vi "Model - DeInit.vi"(8 "error in (no error)":errorcluster, 11 "View Model":T1) -> (0 "error out":errorcluster)   [LabVIEW 2017]
doc: "Deletes all DVR and Destroy all user events from View Model"
uses:
  Controls/View Model.ctl
  Configuration Database/Controls/Config Model.ctl
  Configuration Database/Controls/Config Commands.ctl
  Configuration Database/Controls/Congif Data.ctl
  Controls/Shared Model.ctl
  Error Handler/Controls/Error Model.ctl
  Error Handler/Controls/Error Data.ctl
  Error Handler/Controls/Error Type.ctl
  Car Wash Controller/Controls/Car Wash Model.ctl
  Car Wash Controller/Controls/Controller Overhead.ctl
  Car Wash Controller/Controls/Vehicle Location.ctl
  Car Wash Controller/Controls/Car Wash States.ctl
  Car Wash Controller/Controls/CarWash CMD.ctl
  Views/Wash Display Console View/Controls/Car Wash Indicators.ctl
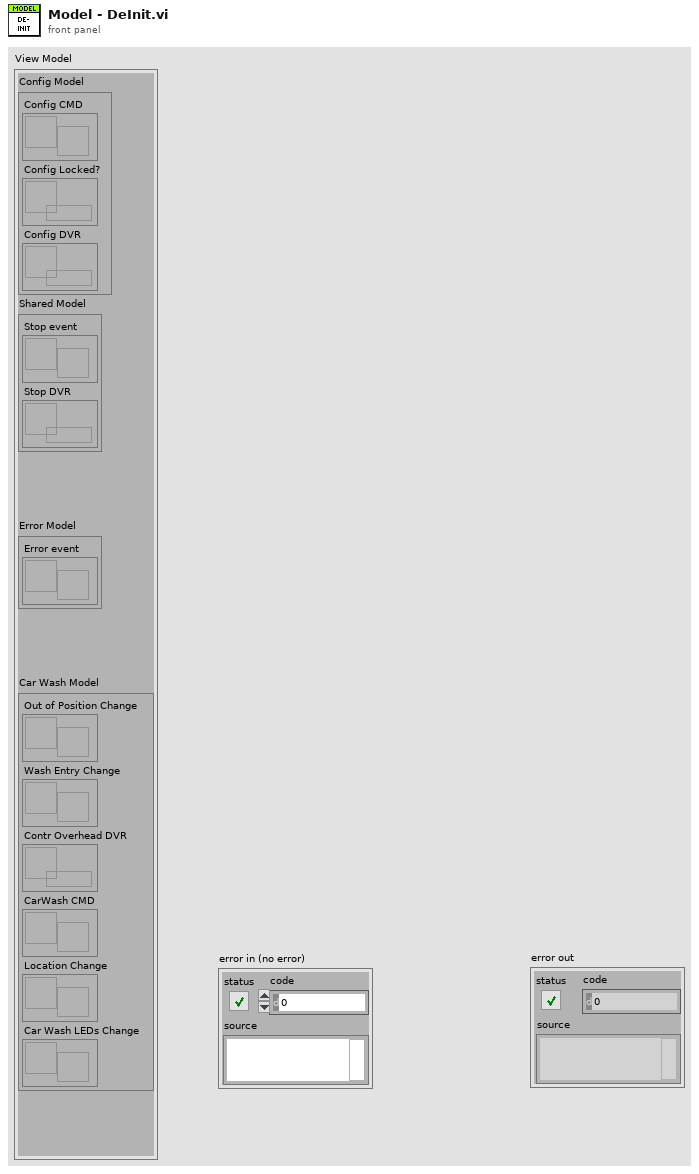
[diagram p1: front panel]
types:
  T1 = typedef "View Model.ctl" = cluster{"Config Model":T2, "Shared Model":T3, "Error Model":T4, "Car Wash Model":T5}
  T2 = typedef "Config Model.ctl" = cluster{"Config CMD":refnum<user-event>, "Config Locked?":refnum<data-value>, "Config DVR":refnum<data-value>}
  T3 = typedef "Shared Model.ctl" = cluster{"Stop event":refnum<user-event>, "Stop DVR":refnum<data-value>}
  T4 = typedef "Error Model.ctl" = cluster{"Error event":refnum<user-event>}
  T5 = typedef "Car Wash Model.ctl" = cluster{"Out of Position Change":refnum<user-event>, "Wash Entry Change":refnum<user-event>, "Contr Overhead DVR":refnum<data-value>, "CarWash CMD":refnum<user-event>, "Location Change":refnum<user-event>, "Car Wash LEDs Change":refnum<user-event>}
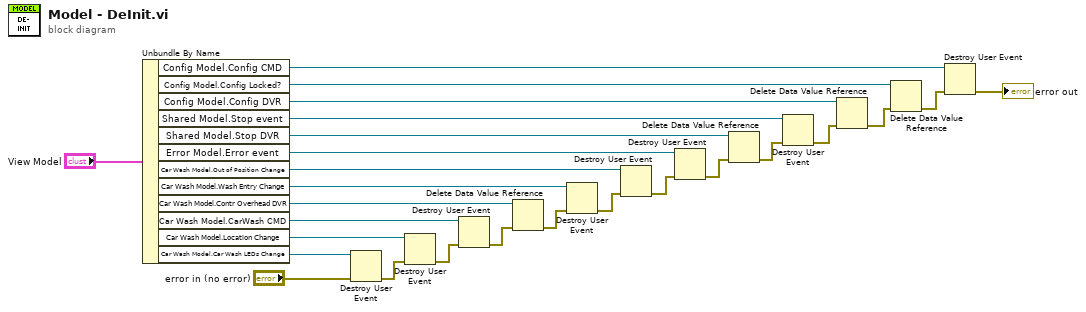
[diagram p0: block diagram]
diagram:
  n1 = Unbundle By Name("View Model") -> ("Config Model.Config CMD"=w3:refnum<user-event>, "Config Model.Config Locked?"=w5:refnum<data-value>, "Config Model.Config DVR"=w7:refnum<data-value>, "Shared Model.Stop event"=w9:refnum<user-event>, "Shared Model.Stop DVR"=w11:refnum<data-value>, "Error Model.Error event"=w13:refnum<user-event>, "Car Wash Model.Out of Position Change"=w15:refnum<user-event>, "Car Wash Model.Wash Entry Change"=w17:refnum<user-event>, "Car Wash Model.Contr Overhead DVR"=w19:refnum<data-value>, "Car Wash Model.CarWash CMD"=w21:refnum<user-event>, "Car Wash Model.Location Change"=w23:refnum<user-event>, "Car Wash Model.Car Wash LEDs Change"=w25:refnum<user-event>)
  n2 = Destroy User Event(user event=w25, error in="error in (no error)") -> (error out=w22:errorcluster)
  n3 = Destroy User Event(user event=w23, error in=w22) -> (error out=w20:errorcluster)
  n4 = Destroy User Event(user event=w21, error in=w20) -> (error out=w18:errorcluster)
  n5 = Delete Data Value Reference(data value reference=w19, error in=w18) -> (error out=w16:errorcluster)  [unwired: 1 out]
  n6 = Destroy User Event(user event=w17, error in=w16) -> (error out=w14:errorcluster)
  n7 = Destroy User Event(user event=w15, error in=w14) -> (error out=w12:errorcluster)
  n8 = Destroy User Event(user event=w13, error in=w12) -> (error out=w10:errorcluster)
  n9 = Delete Data Value Reference(data value reference=w11, error in=w10) -> (error out=w8:errorcluster)  [unwired: 1 out]
  n10 = Destroy User Event(user event=w9, error in=w8) -> (error out=w6:errorcluster)
  n11 = Delete Data Value Reference(data value reference=w7, error in=w6) -> (error out=w4:errorcluster)  [unwired: 1 out]
  n12 = Delete Data Value Reference(data value reference=w5, error in=w4) -> (error out=w2:errorcluster)  [unwired: 1 out]
  n13 = Destroy User Event(user event=w3, error in=w2) -> (error out=→"error out":errorcluster)
